vi "Gyro Testing.vi"   [LabVIEW 2014]
uses:
  <vilib>/Rock Robotics/SystemInterfaces/AI/FPGA_AIGyroChannel.ctl
  Global Variables/Refnum Names.vi
  <vilib>/Rock Robotics/Network Tables/SD Read Number.vi
types:
  T1 = typedef "FPGA_AIGyroChannel.ctl" = enum8{"AI 0", "AI 1", "Invalid"}
  T2 = typedef "WPI_GyroDevRef.ctl" = cluster{"DevStatus":errorcluster, "Analog Module":T3, "Analog Channel":T4, "Offset":dbl, "Gain (VoltsPerDegree/Second)":dbl}
  T3 = typedef "FPGA_TypedefAnalogModule.ctl" = enum16{"Controller 1"}
  T4 = typedef "FPGA_AIChannel.ctl" = enum8{"AI 0", "AI 1", "AI 2", "AI 3", "AI MXP 0", "AI MXP 1", "AI MXP 2", "AI MXP 3", "Invalid"}
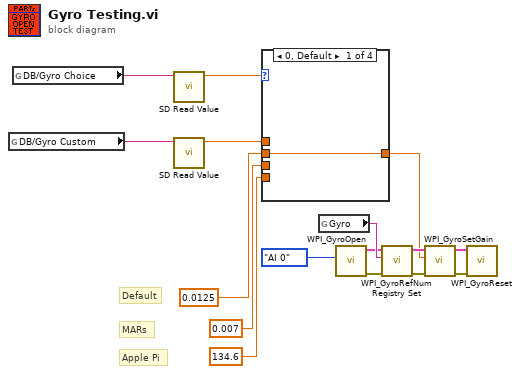
[diagram p0: block diagram]
diagram:
  # "Default"
  # "MARs"
  # "Apple Pi"
  n1 = global read "Refnum Names.vi" "DB/Gyro Custom"() -> (w6:string)
  n2 = global read "Refnum Names.vi" "DB/Gyro Choice"() -> (w8:string)
  n3 = call-poly <vilib>:"SD Read Value.vi"("Name"=w8) -> ("Numeric"=w7:dbl)  [unwired: 8 in, 2 out]
  n4 = call-poly <vilib>:"SD Read Value.vi"("Name"=w6) -> ("Numeric"=w1:dbl)  [unwired: 8 in, 2 out]
  n5 = case shown="0, Default" w7 {
    tunnel: [w17 w18 w19 w20] -> w4
    tunnel: 0.0125 ("Gain (VoltsPerDegree/Second)") -> [w17 _ _ _]
    tunnel: 0.007 ("Gain (VoltsPerDegree/Second)") -> [_ w18 _ _]
    tunnel: 134.6 ("Calibrated Center Voltage") -> [_ _ w19 _]
    tunnel: w1 -> [_ _ _ w20]
    frame 0, Default {
    }
    frame 1 {
    }
    frame 2 {
    }
    frame 3 {
    }
  }
  n6 = global read "Refnum Names.vi" "Gyro"() -> (w15:string)
  n7 = call <vilib>:"WPI_GyroOpen.vi"("Analog Channel"=FPGA_AIGyroChannel."AI 0") -> ("error out"=w9:errorcluster, "GyroDevRef"=w10:T2)  [unwired: 8 in, 1 out]
  n8 = call <vilib>:"WPI_GyroRefNum Registry Set.vi"("error in (no error)"=w9, "refnum name"=w15, "GyroDevRef"=w10) -> ("error out"=w11:errorcluster, "GyroDevRef"=w12:T2)  [unwired: 7 in]
  n9 = call <vilib>:"WPI_GyroSetGain.vi"("error in (no error)"=w11, "Gain (VoltsPerDegree/Second)"=w4, "GyroDevRef"=w12) -> ("error out"=w13:errorcluster, "GyroDevRef"=w14:T2)  [unwired: 7 in]
  n10 = call <vilib>:"WPI_GyroReset.vi"("error in (no error)"=w13, "GyroDevRef"=w14) -> ()  [unwired: 8 in, 2 out]
